vi "Write Input Power Initialized.vi"(8 "error in (no error)":errorcluster, 10 "Input Power Initialized":bool, 11 "Test Group in":refnum<class "Test Group.lvclass">) -> (0 "error out":errorcluster, 3 "Test Group out":refnum<class "Test Group.lvclass">)   [LabVIEW 2016, in "Test Group Manager.lvlib" / "Test Group.lvclass"]
uses:
  Test Group.lvclass
  Test Group.lvclass/Test Group.ctl
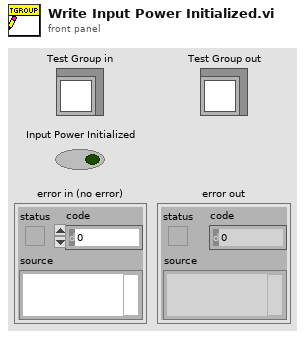
[diagram p1: front panel]
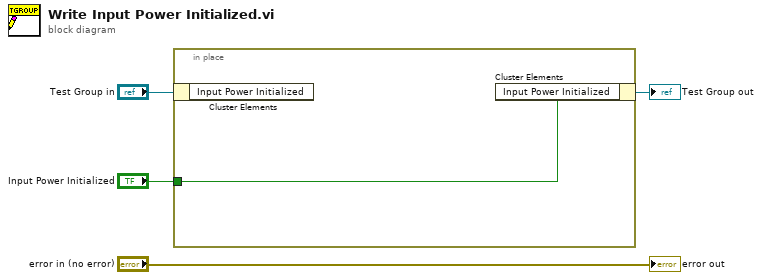
[diagram p0: block diagram]
diagram:
  n1 = in-place {
    in-place-border: "Input Power Initialized" -> [w5]
    n2 = in-place-cluster #1("Test Group in") -> ()  [unwired: 1 out]
    n3 = in-place-cluster #1("Input Power Initialized"=w5) -> (→"Test Group out":refnum<class "Test Group.lvclass">)
  }
  "error out" <- "error in (no error)"
